vi "DBM STD File Open.vi"(6 "TBCALSTD":refnum<vi>, 7 "교정일자":refnum<vi>, 8 "에러 입력":errorcluster caption="에러 입력(에러 없음)", 9 "close report? (T)":bool=TRUE caption="리포트 닫기?(참)", 10 "index (0)":i32, 11 "report out":refnum<class "NI_report.lvclass"> caption="리포트 입력") -> (0 "에러 출력":errorcluster, 1 "등록번호":string, 4 "Cal Date ok?":bool, 5 "STDDB ok?":bool)   [LabVIEW 2020]
uses:
  <vilib>/Utility/NIReport.llb/NI_report.lvclass
  Controls/Cmd_Read Query.ctl
  Controls/Clst_Query Info.ctl
  <vilib>/addons/_office/excel.llb/Excel Get Data ([str]).vi
  Public/Polymorph/Rmv Empt Arr_2D Str.vi
  Public/Polymorph/Array Dedup_1D Str.vi
  Public/Polymorph/Cell Space_Table.vi
  <vilib>/addons/_office/NI_ReportGenerationToolkit.lvlib
  <vilib>/Utility/NIReport.llb/Excel/NI_Excel.lvclass
  <vilib>/addons/database/NI_Database_API.lvlib
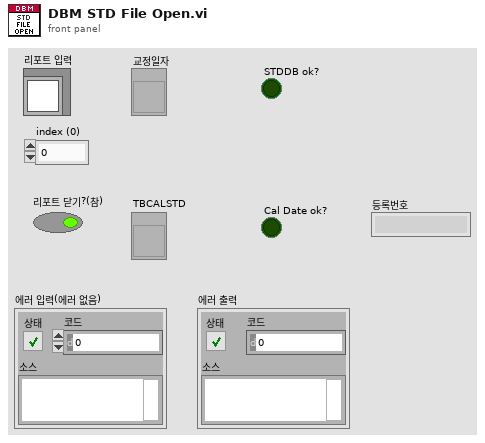
[diagram p1: front panel]
types:
  T1 = typedef "Cmd_Read Query.ctl" = enum16{"교정자 이름 얻기", "인증교정자 얻기", "기술책임자 얻기", "기책부책 얻기", "등록번호 얻기", "등록정보 얻기", "업체정보 얻기", "교정일자(CAMAS) 얻기", "교정일자(CALSTD) 얻기", "교정환경 얻기", "교정절차서 목록 얻기", "교정절차서명 얻기", "교정절차 목록얻기", "교정절차 얻기", "PROC 교정절차 얻기", "PROC SPEC 얻기", "교정절차(Func별) 얻기", "교정절차(Func_ext별) 얻기", "기관코드 얻기", "교정기능(세부분류) 얻기", "교정기능(모델) 얻기", "교정기능 목록 얻기", "교정기능 명칭 얻기", "교정기능 항목명칭 얻기", "DB (사용기준기) 얻기", "DB (기준기이름) 얻기", "DB (기준기이름목록) 얻기", "DB (기준기목록) 얻기", "DB (기준기값) 얻기", "DB (CMC) 얻기", "DB (FUNC) 얻기", "DB (CALNAME) 얻기", "DB (STDNAME) 얻기", "DB (SPEC) 얻기", "모델(항목전체) 얻기", "모델(최대범위) 얻기", "모델(최소범위) 얻기", "모델(최대최소) 얻기", "모델(범위조건) 얻기", "모델(등록요청) 얻기", "모델(형식별) 얻기", "모델(조건별) 얻기", "모델(모델검색) 얻기", "세부분류 목록 얻기", "기준기등록리스트 얻기", "STD Cal Date Check", "DB등록일자 얻기", "적용항목 얻기", "기타정보 얻기", "기준기요청 얻기", "서버버전 얻기"}
  T2 = typedef "Clst_Query Info.ctl" = cluster{"사번":string, "등록번호":string, "업체명":string, "세부분류코드":string, "형식":string, "기기번호":string, "FUNC":string, "FUNC_EXT":string, "옵션":string, "추가문자열":string, "일자":string, "배열 1":string[], "배열 2":string[], "항목명":string, "문자열":string, "이름":string}
  T3 = cluster{"position (excel)":cluster{"row":i32, "column":i32}, "name (excel)":string, "bookmark (word)":string}
  T4 = typedef "NI_Database_API.lvlib/Conn ObjectReference.ctl" = refnum<k1>
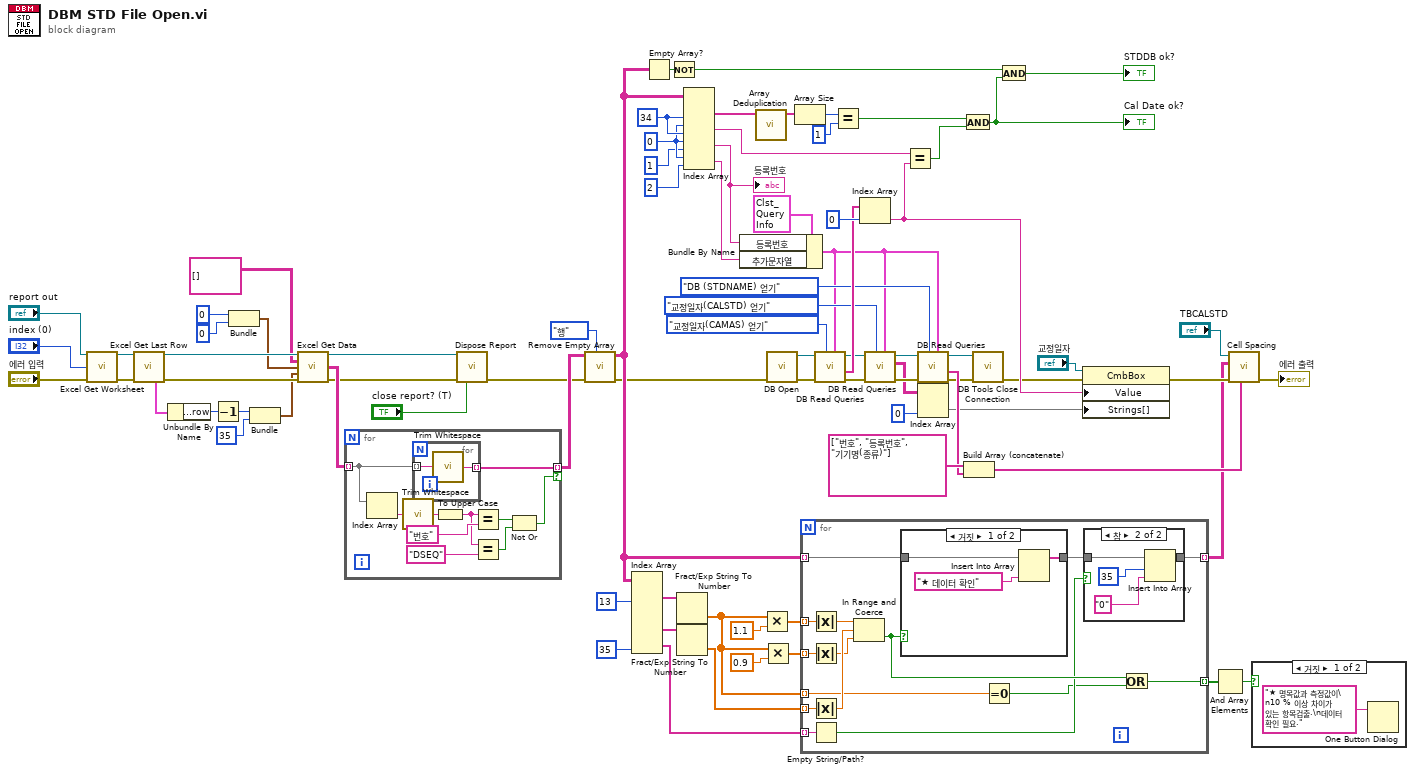
[diagram p0: block diagram]
diagram:
  w28 = 0 ("비활성화된 인덱스 (행)")
  w30 = 34 ("비활성화된 인덱스 (열)")
  n1 = call <vilib>:"Excel Get Worksheet.vi"("report in"="report out", "worksheet index (0)"="index (0)", "error in (no error)"="에러 입력") -> ("report out"=w2:refnum<class "NI_report.lvclass">, "error out"=w3:errorcluster)  [unwired: 11 in]
  n2 = call <vilib>:"Excel Get Last Row.vi"("report in"=w2, "error in (no error)"=w3) -> ("report out"=w67:refnum<class "NI_report.lvclass">, "MS Office parameters out"=w68:T3, "error out"=w66:errorcluster)  [unwired: 11 in]
  n3 = Unbundle By Name(w68) -> ("position (excel).row"=w61:i32)
  n4 = Decrement(x=w61) -> (x-1=w48:i32)
  n5 = Bundle(0, 0) -> (w62:cluster{i32, i32})  [unwired: 1 in]
  n6 = Bundle(w48, 35) -> (w59:cluster{i32, i32})  [unwired: 1 in]
  n7 = call-poly <vilib>:"Excel Get Data.vi"("report in"=w67, "data type"=string[][] [], "start (-1, -1)"=w62, "end (-1, -1)"=w59, "error in (no error)"=w66) -> ("report out"=w7:refnum<class "NI_report.lvclass">, "data"=w47:string[][], "error out"=w8:errorcluster)  [unwired: 8 in]
  n8 = for {
    tunnel: w47 -> [w84] mode=indexing
    tunnel: [w83] -> w46 mode=indexing if=w85
    n9 = Index Array(array=w84) -> (element=w92:string)  [unwired: 1 in]
    n10 = call <vilib>:"Trim Whitespace.vi"("string"=w92) -> ("trimmed string"=w90:string)  [unwired: 1 in]
    n11 = for {
      tunnel: w84 -> [w94] mode=indexing
      tunnel: [w93] -> w83 mode=indexing
      n12 = call <vilib>:"Trim Whitespace.vi"("string"=w94) -> ("trimmed string"=w93:string)  [unwired: 1 in]
    }
    n13 = To Upper Case(1:w90) -> (0:w88:string)
    n14 = Equal?(x=w88, y="번호") -> (x = y?=w87:bool)
    n15 = Equal?(x=w88, y="DSEQ") -> (x = y?=w86:bool)
    n16 = Not Or(1:w86, 2:w87) -> (0:w85:bool)
  }
  n17 = call-dynamic "Dispose Report.vi"("report in"=w7, "error in (no error)"=w8, "close report? (T)"="close report? (T)") -> ()  [unwired: 12 in, 1 out]
  n18 = call-poly "Remove Empty Array.vi"("조건"=enum16{"행", "열", "행,열"}."행", "error in (no error)"=w8, "Data in"=w46) -> ("error out"=w14:errorcluster, "Data out"=w51:string[][])  [unwired: 7 in]
  n19 = Index Array(array=w51, index (col) #1=13 ("인덱스"), index (col) #4=35 ("인덱스")) -> (element #1=w57:string[], element #3=w56:string[], element #4=w33:string[])  [unwired: 6 in, 1 out]
  n20 = Empty Array?(array=w51) -> (empty?=w79:bool)
  n21 = Not(x=w79) -> (.not. x?=w80:bool)
  n22 = Fract/Exp String To Number(string=w57) -> (number=w31:dbl[])  [unwired: 3 in, 1 out]
  n23 = Fract/Exp String To Number(string=w56) -> (number=w32:dbl[])  [unwired: 3 in, 1 out]
  n24 = Index Array(array=w51, index (col) #1=w30, index (row) #2=w28, index (col) #2=w30, index (row) #3=w28, index (col) #3=1 ("비활성화된 인덱스 (열)"), index (row) #4=w28, index (col) #4=2 ("비활성화된 인덱스 (열)")) -> (element #1=w29:string[], element #2=w75:string, element #3=w26:string, element #4=w24:string)  [unwired: 1 in]
  "등록번호" <- w26
  n25 = Bundle By Name(cluster=T2 {"사번"="", "등록번호"="", "업체명"="", "세부분류코드"="", "형식"="", "기기번호"="", "FUNC"="", "FUNC_EXT"="", "옵션"="", "추가문자열"="", "일자"="", "배열 1"=[], "배열 2"=[], "항목명"="", "문자열"="", "이름"=""} ("Query info"), "등록번호"=w26, "추가문자열"=w24) -> (w23:T2)
  n26 = call-poly "Array Deduplication.vi"("배열 in"=w29) -> ("배열 out"=w72:string[])  [unwired: 9 in, 1 out]
  n27 = Multiply(x=w31, y=1.1) -> (x*y=w53:dbl[])
  n28 = Multiply(x=w31, y=0.9) -> (x*y=w52:dbl[])
  n29 = call "DB Open.vi"("에러 입력"=w14) -> ("에러 출력"=w13:errorcluster, "참조 번호 출력"=w12:T4)  [unwired: 9 in]
  n30 = Array Size(array=w72) -> (size(s)=w73:i32)
  n31 = for {
    tunnel: w53 -> [w109] mode=indexing
    tunnel: w52 -> [w108] mode=indexing
    tunnel: w32 -> [w107] mode=indexing
    tunnel: w51 -> [w106] mode=indexing
    tunnel: [w100] -> w15 mode=indexing
    tunnel: [w96] -> w49 mode=indexing
    tunnel: w33 -> [w99] mode=indexing
    tunnel: w31 -> [w97] mode=indexing
    n32 = Absolute Value(x=w109) -> (abs(x)=w104:dbl)
    n33 = Absolute Value(x=w108) -> (abs(x)=w102:dbl)
    n34 = Absolute Value(x=w107) -> (abs(x)=w103:dbl)
    n35 = Empty String/Path?(string/path=w99) -> (empty?=w98:bool)
    n36 = In Range and Coerce(upper limit=w104, x=w103, lower limit=w102) -> (In Range?=w105:bool)  [unwired: 1 out]
    n37 = case shown="거짓" w105 {
      tunnel: w106 -> [w117 w118]
      tunnel: [w116 w118] -> w101
      frame False {
        n38 = Insert Into Array(array=w117, new element="★ 데이터 확인") -> (w116:string[])  [unwired: 1 in]
      }
      frame True {
      }
    }
    n39 = Equal To 0?(x=w97) -> (x = 0?=w95:bool)
    n40 = case shown="참" w98 {
      tunnel: [w110 w114] -> w100
      tunnel: w101 -> [w110 w112]
      frame False {
      }
      frame True {
        n41 = Insert Into Array(array=w112, index=35 ("인덱스"), new element="0" ("새 원소/부분배열")) -> (w114:string[])
      }
    }
    n42 = Or(x=w105, y=w95) -> (x .or. y?=w96:bool)
  }
  n43 = call "DB Read Queries.vi"("Query info"=w23, "Query Command"=Cmd_Read_Query."교정일자(CAMAS) 얻기", "에러 입력(에러 없음)"=w13, "참조 번호 입력"=w12) -> ("에러 출력"=w41:errorcluster, "Data (0번행)"=w70:string[], "참조 번호 출력"=w40:T4)  [unwired: 3 in, 2 out]
  n44 = Equal?(x=w73, y=1) -> (x = y?=w77:bool)
  n45 = Index Array(array=w70, index=0 ("인덱스")) -> (element=w21:string)
  n46 = call "DB Read Queries.vi"("Query info"=w23, "Query Command"=Cmd_Read_Query."교정일자(CALSTD) 얻기", "에러 입력(에러 없음)"=w41, "참조 번호 입력"=w40) -> ("에러 출력"=w39:errorcluster, "Data"=w36:string[][], "참조 번호 출력"=w38:T4)  [unwired: 3 in, 2 out]
  n47 = Equal?(x=w75, y=w21) -> (x = y?=w76:bool)
  n48 = call "DB Read Queries.vi"("Query info"=w23, "Query Command"=Cmd_Read_Query."DB (STDNAME) 얻기", "에러 입력(에러 없음)"=w39, "참조 번호 입력"=w38) -> ("에러 출력"=w10:errorcluster, "Data (0번행)"=w42:string[], "참조 번호 출력"=w11:T4)  [unwired: 3 in, 2 out]
  n49 = Index Array(array=w36, index (col)=0 ("인덱스 (행)")) -> (element=w20:string[])  [unwired: 1 in]
  n50 = And(x=w77, y=w76) -> (x .and. y?=w81:bool)
  "Cal Date ok?" <- w81
  n51 = Build Array (concatenate)(string[] ["번호", "등록번호", "기기명(종류)"], w42) -> (w16:string[])
  n52 = call <vilib>:"DB Tools Close Connection.vi"("error in (no error)"=w10, "connection reference"=w11) -> ("error out"=w9:errorcluster)  [unwired: 5 in]
  n53 = And(x=w80, y=w81) -> (x .and. y?=→"STDDB ok?":bool)
  n54 = property on="프로퍼티 노드" class="CmbBox"(reference="교정일자", error in=w9, "Value"=w21, "Strings[]"=w20) -> (error out=w19:errorcluster)  [unwired: 1 out]
  n55 = And Array Elements(Boolean array=w49) -> (logical AND=w50:bool)
  n56 = call-poly "Cell Spacing.vi"("Col Header in"=w16, "error in"=w19, "Data in"=w15, "테이블 참조 in"="TBCALSTD") -> ("error out"=→"에러 출력":errorcluster)  [unwired: 5 in, 2 out]
  n57 = case shown="거짓" w50 {
    frame False {
      n58 = One Button Dialog(message="★ 명목값과 측정값이\n10 % 이상 차이가 있는 항목검출.\n데이터 확인 필요.") -> ()  [unwired: 1 in, 1 out]
    }
    frame True {
    }
  }
